vi "Initialize_TIGER_module.vi"() -> (0 "error out":errorcluster, 3 "Status readout":string="Already in external (NI-DAQ)")   [LabVIEW 2016]
uses:
  <vilib>/Instr/_visa.llb/VISA Configure Serial Port (Instr).vi
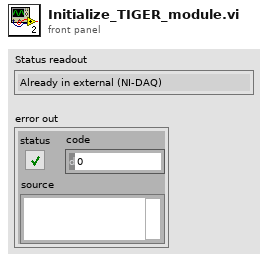
[diagram p1: front panel]
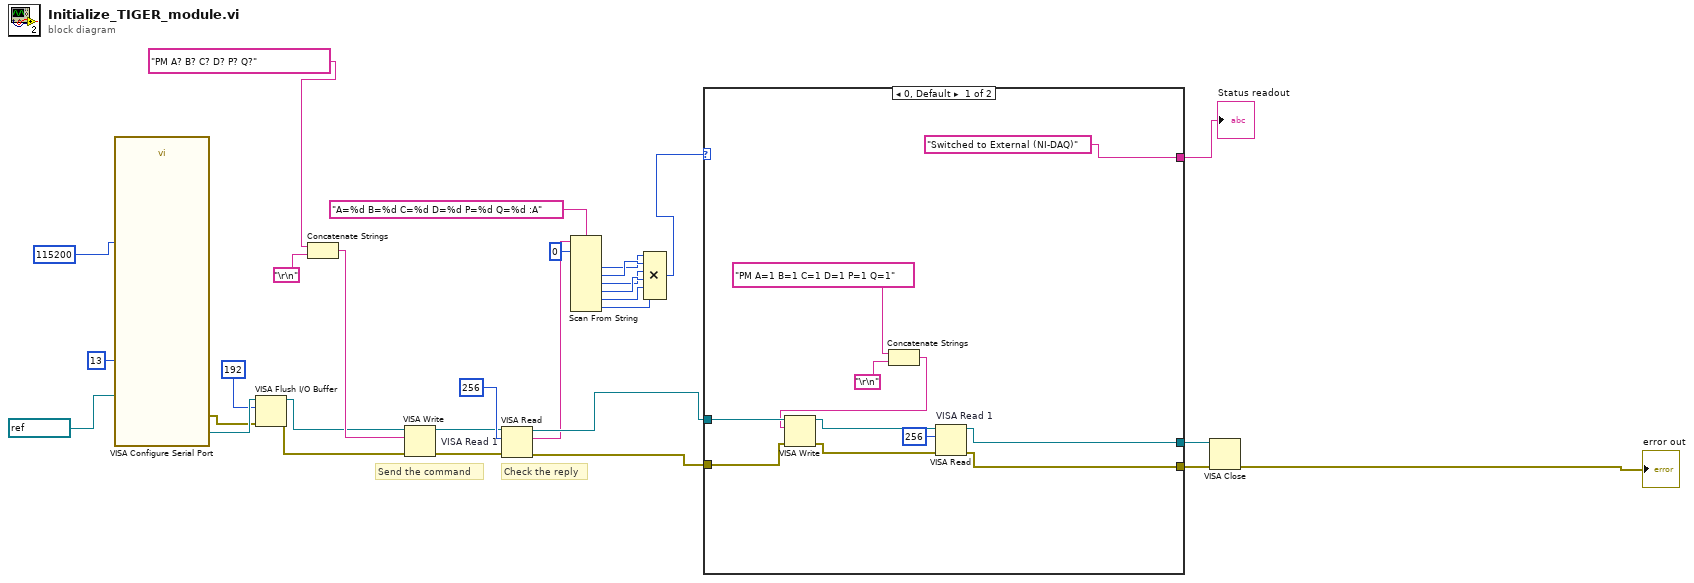
[diagram p0: block diagram]
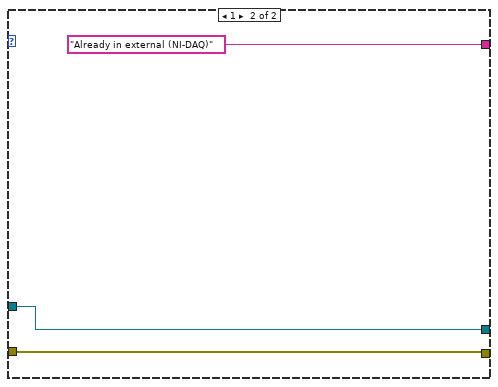
[diagram p2: hidden frame]
diagram:
  # "Check the reply"
  # "Send the command"
  n1 = call-poly "VISA Configure Serial Port"("VISA resource name"=refnum<visa-resource-name> "COM6", "termination char\n(0xA = '\\n' = LF)"=u8 13 ("termination char\n(0xA = '\\n' = LF)"), "baud rate (9600)"=u32 115200) -> ("VISA resource name out"=w8:refnum<visa-resource-name>, "error out"=w7:errorcluster)  [unwired: 4 in, 7 out]
  n2 = VISA Flush I/O Buffer(VISA resource name=w8, mask (16)=u16 192 ("Mask"), error in (no error)=w7) -> (VISA resource name out=w5:refnum<visa-resource-name>, error out=w4:errorcluster)
  n3 = Concatenate Strings("PM A? B? C? D? P? Q?" ("write buffer"), "\r\n") -> (w13:string)
  n4 = VISA Write(VISA resource name=w5, write buffer=w13, error in (no error)=w4) -> (VISA resource name out=w2:refnum<visa-resource-name>, error out=w1:errorcluster)  [unwired: 1 out]
  n5 = VISA Read "VISA Read 1"(VISA resource name=w2, byte count=u32 256, error in (no error)=w1) -> (VISA resource name out=w26:refnum<visa-resource-name>, read buffer=w15:string, error out=w27:errorcluster)  [unwired: 1 out]
  n6 = Scan From String(format string="A=%d B=%d C=%d D=%d P=%d Q=%d :A", input string=w15, initial scan location=u32 0) -> (output 1=w18:i32, output 2=w19:i32, output 3=w20:i32, output 4=w21:i32, output 5=w22:i32, output 6=w23:i32)  [unwired: 7 in, 3 out]
  n7 = Compound Arithmetic op=MULTIPLY(w18, w19, w20, w21, w22, w23) -> (w24:i32)
  n8 = case shown="0, Default" w24 {
    tunnel: w26 -> [w41 w44]
    tunnel: w27 -> [w39 w43]
    tunnel: [w36 w43] -> w28
    tunnel: [w35 w44] -> w29
    tunnel: ["Switched to External (NI-DAQ)" "Already in external (NI-DAQ)"] -> w30
    frame 0, Default {
      n9 = Concatenate Strings("PM A=1 B=1 C=1 D=1 P=1 Q=1" ("write buffer"), "\r\n") -> (w32:string)
      n10 = VISA Write(VISA resource name=w41, write buffer=w32, error in (no error)=w39) -> (VISA resource name out=w40:refnum<visa-resource-name>, error out=w38:errorcluster)  [unwired: 1 out]
      n11 = VISA Read "VISA Read 1"(VISA resource name=w40, byte count=u32 256, error in (no error)=w38) -> (VISA resource name out=w35:refnum<visa-resource-name>, error out=w36:errorcluster)  [unwired: 2 out]
    }
    frame 1 {
    }
  }
  "Status readout" <- w30
  n12 = VISA Close(VISA resource name=w29, error in (no error)=w28) -> (error out=→"error out":errorcluster)
